vi "SymbolEnumToIndex.vi"(11 "symbol enum":T1=enum."Float") -> (3 "ItemSyms":i32)   [LabVIEW 2019, in "BlueVariantView.lvlib"]
uses:
  BlueVariantView.lvlib
  Symbol.ctl
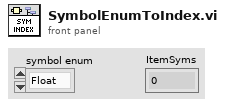
[diagram p1: front panel]
types:
  T1 = typedef "BlueVariantView.lvlib/Symbol.ctl" = enum16{"None", "Cluster-brown", "Cluster-yellow", "Cluster-black", "Cluster-pink", "Array", "Float", "Int", "Bool", "String", "Enum", "Object", "Map", "Set", "Refnum", "Variant", "Path", "Picture", "Waveform", "Timestamp", "Digital Waveform", "Fixed Point"}
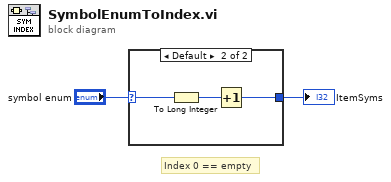
[diagram p0: block diagram]
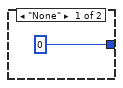
[diagram p2: hidden frame]
diagram:
  # "Index 0 == empty"
  n1 = case shown="Default" "symbol enum" {
    selector: "symbol enum" -> [_ w6]
    tunnel: [0 w5] -> w1
    frame "None" {
    }
    frame Default {
      n2 = To Long Integer(number=w6) -> (32bit integer=w4:i32)
      n3 = Increment(x=w4) -> (x+1=w5:i32)
    }
  }
  "ItemSyms" <- w1
